vi "ex2.vi"() -> ()   [LabVIEW 2022 SP3]
uses:
  #typedef_ex2_states.ctl
panel:
  out "Pressed numbers":string
  in  "Button 9":bool
  in  "Button 6":bool
  in  "Button 8":bool
  in  "Button 5":bool
  in  "Button 7":bool
  in  "Button 4":bool
  in  "Button 3":bool
  in  "Button 2":bool
  in  "Button 1":bool
  in  "Button 0":bool
  in  "Reset Record":bool
  in  "Stop Program":bool
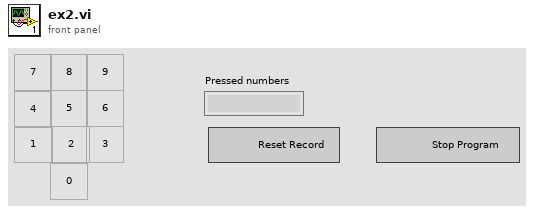
[diagram p1: front panel]
types:
  T1 = typedef "#typedef_ex2_states.ctl" = enum16{"Idle", "9 was chosen", "8 was chosen", "7 was chosen", "6 was chosen", "5 was chosen", "4 was chosen", "3 was chosen", "2 was chosen", "1 was chosen", "0 was chosen", "Refresh GUI", "Reset Record", "Exit", "Eror State"}
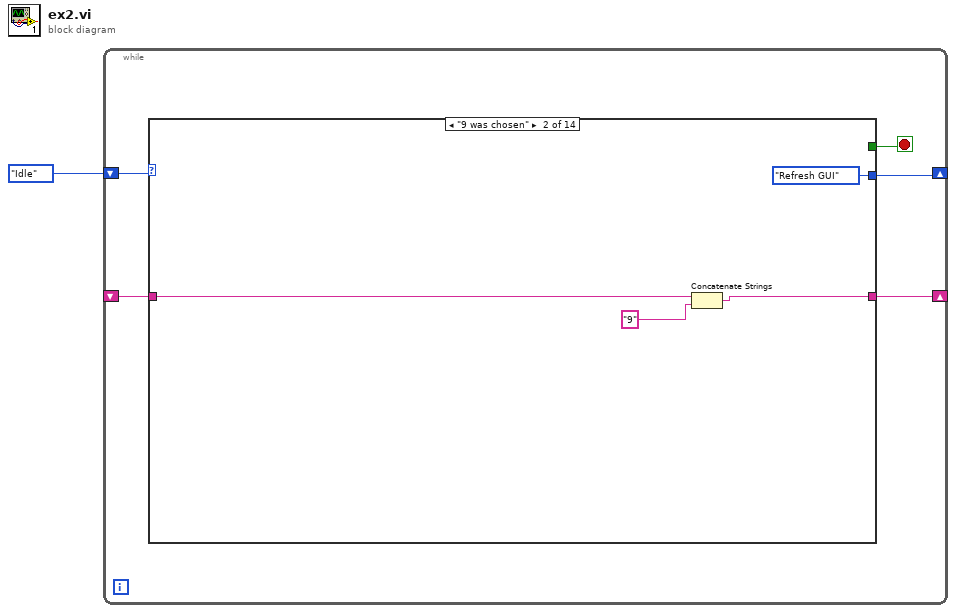
[diagram p0: block diagram]
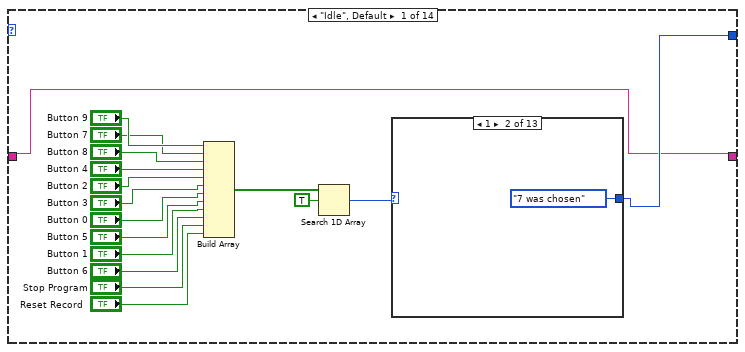
[diagram p2: hidden frame]
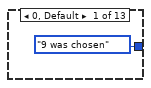
[diagram p3: hidden frame]
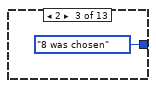
[diagram p4: hidden frame]
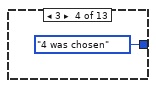
[diagram p5: hidden frame]
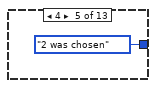
[diagram p6: hidden frame]
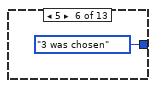
[diagram p7: hidden frame]
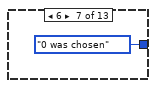
[diagram p8: hidden frame]
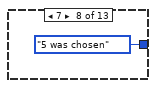
[diagram p9: hidden frame]
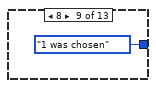
[diagram p10: hidden frame]
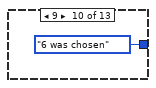
[diagram p11: hidden frame]
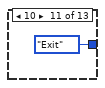
[diagram p12: hidden frame]
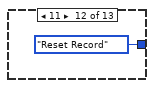
[diagram p13: hidden frame]
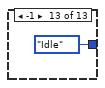
[diagram p14: hidden frame]
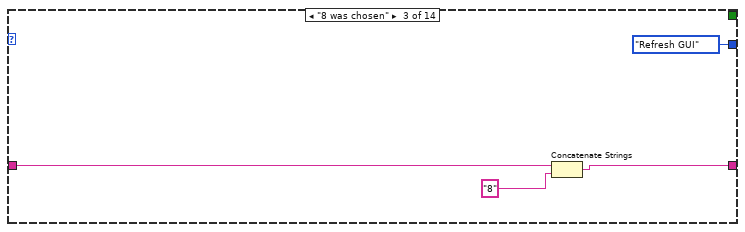
[diagram p15: hidden frame]
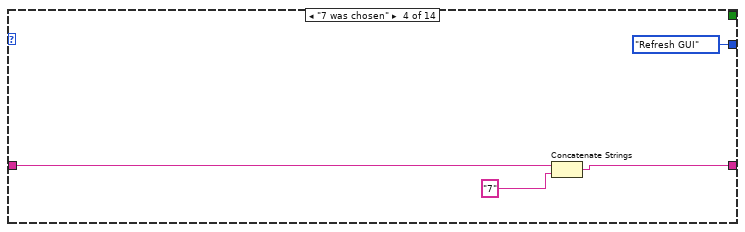
[diagram p16: hidden frame]
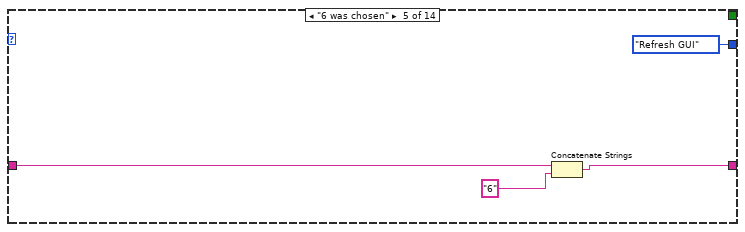
[diagram p17: hidden frame]
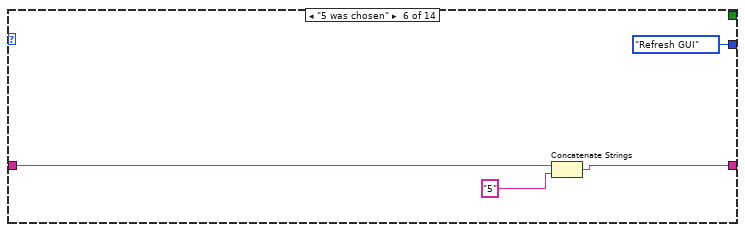
[diagram p18: hidden frame]
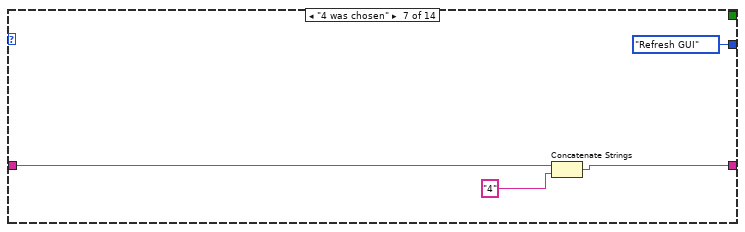
[diagram p19: hidden frame]
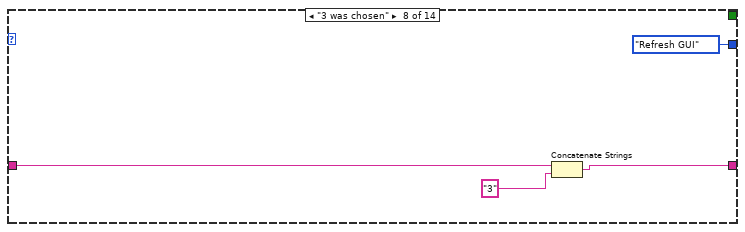
[diagram p20: hidden frame]
diagram:
  n1 = while {
    shift-right: [w4] -> _
    shift-left: #typedef_ex2_states."Idle" ("Enum") -> [w5]
    shift-right: [w3] -> _
    shift-left: _ -> [w2]
    stop <- w6 stop-if-true
    n2 = case shown="\"9 was chosen\"" w5 {
      tunnel: [w8 #typedef_ex2_states."Refresh GUI" ("Enum") #typedef_ex2_states."Refresh GUI" ("Enum") #typedef_ex2_states."Refresh GUI" ("Enum") #typedef_ex2_states."Refresh GUI" ("Enum") #typedef_ex2_states."Refresh GUI" ("Enum") #typedef_ex2_states."Refresh GUI" ("Enum") #typedef_ex2_states."Refresh GUI" ("Enum") #typedef_ex2_states."Refresh GUI" ("Enum") #typedef_ex2_states."Refresh GUI" ("Enum") #typedef_ex2_states."Refresh GUI" ("Enum") #typedef_ex2_states."Exit" ("Enum") #typedef_ex2_states."Refresh GUI" ("Enum") #typedef_ex2_states."Idle" ("Enum")] -> w4
      tunnel: [_ _ _ _ _ _ _ _ _ _ _ TRUE _ _] -> w6
      tunnel: [w7 w38 w42 w46 w50 w54 w58 w62 w66 w70 w74 w77 w80 w84] -> w3
      tunnel: w2 -> [w7 w40 w44 w48 w52 w56 w60 w64 w68 w72 w76 w77 w82 w84]
      frame "Idle", Default {
        n3 = Build Array("Button 9", "Button 7", "Button 8", "Button 4", "Button 2", "Button 3", "Button 0", "Button 5", "Button 1", "Button 6", "Stop Program", "Reset Record") -> (w11:bool[])
        n4 = Search 1D Array(1D array=w11, element=TRUE) -> (index of element=w9:i32)  [unwired: 1 in]
        n5 = case shown="1" w9 {
          tunnel: [#typedef_ex2_states."9 was chosen" ("Enum") #typedef_ex2_states."7 was chosen" ("Enum") #typedef_ex2_states."8 was chosen" ("Enum") #typedef_ex2_states."4 was chosen" ("Enum") #typedef_ex2_states."2 was chosen" ("Enum") #typedef_ex2_states."3 was chosen" ("Enum") #typedef_ex2_states."0 was chosen" ("Enum") #typedef_ex2_states."5 was chosen" ("Enum") #typedef_ex2_states."1 was chosen" ("Enum") #typedef_ex2_states."6 was chosen" ("Enum") #typedef_ex2_states."Exit" ("Enum") #typedef_ex2_states."Reset Record" ("Enum") #typedef_ex2_states."Idle" ("Enum")] -> w8
          frame 0, Default {
          }
          frame 1 {
          }
          frame 2 {
          }
          frame 3 {
          }
          frame 4 {
          }
          frame 5 {
          }
          frame 6 {
          }
          frame 7 {
          }
          frame 8 {
          }
          frame 9 {
          }
          frame 10 {
          }
          frame 11 {
          }
          frame -1 {
          }
        }
      }
      frame "9 was chosen" {
        n6 = Concatenate Strings(w40, "9" ("Pressed numbers")) -> (w38:string)
      }
      frame "8 was chosen" {
        n7 = Concatenate Strings(w44, "8" ("Pressed numbers")) -> (w42:string)
      }
      frame "7 was chosen" {
        n8 = Concatenate Strings(w48, "7" ("Pressed numbers")) -> (w46:string)
      }
      frame "6 was chosen" {
        n9 = Concatenate Strings(w52, "6" ("Pressed numbers")) -> (w50:string)
      }
      frame "5 was chosen" {
        n10 = Concatenate Strings(w56, "5" ("Pressed numbers")) -> (w54:string)
      }
      frame "4 was chosen" {
        n11 = Concatenate Strings(w60, "4" ("Pressed numbers")) -> (w58:string)
      }
      frame "3 was chosen" {
        n12 = Concatenate Strings(w64, "3" ("Pressed numbers")) -> (w62:string)
      }
      frame "2 was chosen" {
        n13 = Concatenate Strings(w68, "2" ("Pressed numbers")) -> (w66:string)
      }
      frame "1 was chosen" {
        n14 = Concatenate Strings(w72, "1" ("Pressed numbers")) -> (w70:string)
      }
      frame "0 was chosen" {
        n15 = Concatenate Strings(w76, "0" ("Pressed numbers")) -> (w74:string)
      }
      frame "Exit" {
      }
      frame "Reset Record" {
        n16 = Replace Substring(5:w82) -> (0:w80:string)  [unwired: 3 in, 1 out]
      }
      frame "Refresh GUI" {
        "Pressed numbers" <- w84
      }
    }
  }
